vi "Read Enumerated Resources.vi"(8 "error in (no error)":errorcluster, 10 "Refresh":bool=TRUE, 11 "AbstractResourceEnumerator in":refnum<class "AbstractResourceEnumerator.lvclass">) -> (0 "error out":errorcluster, 2 "Enumerated Resources":T1[](array[typedef]), 3 "AbstractResourceEnumerator out":refnum<class "AbstractResourceEnumerator.lvclass">)   [LabVIEW 2023, in "HAF.lvlib" / "AbstractResourceEnumerator.lvclass"]
doc: "Returns the collection of resources connected to the system. The collection can be refreshed before return. If the collection is empty, resources will always be enumerated regardless of the passed indicator."
uses:
  AbstractResourceEnumerator.lvclass
  AbstractResourceEnumerator.lvclass/AbstractResourceEnumerator.ctl
  Resource Structure.ctl
  HAF.lvlib
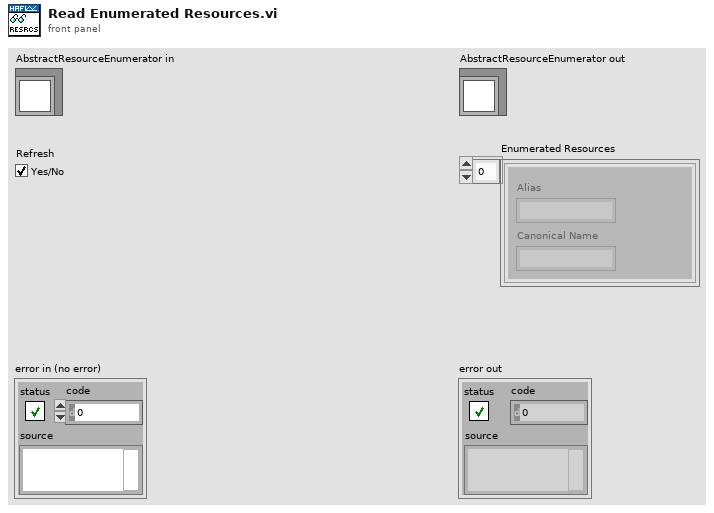
[diagram p1: front panel]
types:
  T1 = typedef "HAF.lvlib/Resource Structure.ctl" = cluster{"Alias":string, "Canonical Name":string}
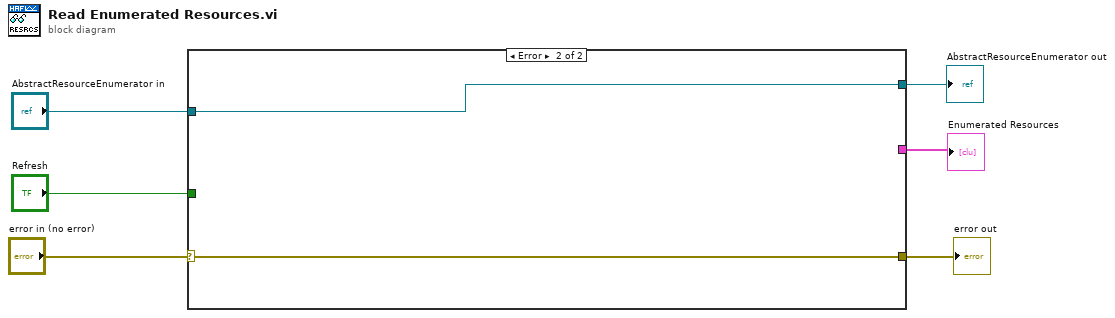
[diagram p0: block diagram]
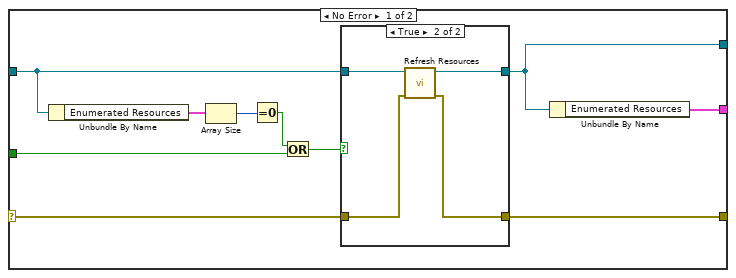
[diagram p2: hidden frame]
diagram:
  n1 = case shown="Error" "error in (no error)" {
    selector: "error in (no error)" -> [w10 w23]
    tunnel: [w9 w23] -> w5
    tunnel: [w8 w24] -> w3
    tunnel: "AbstractResourceEnumerator in" -> [w11 w24]
    tunnel: "Refresh" -> [w13 _]
    tunnel: [w7 _] -> w1
    frame No Error {
      n2 = Unbundle By Name(w11) -> ("Enumerated Resources"=w16:T1[])
      n3 = Array Size(array=w16) -> (size(s)=w15:i32)
      n4 = Equal To 0?(x=w15) -> (x = 0?=w14:bool)
      n5 = Or(x=w14, y=w13) -> (x .or. y?=w12:bool)
      n6 = case shown="True" w12 {
        tunnel: w11 -> [w18 w22]
        tunnel: w10 -> [w17 w20]
        tunnel: [w18 w21] -> w8
        tunnel: [w17 w19] -> w9
        frame False {
        }
        frame True {
          n7 = call-dynamic "Refresh Resources.vi"("error in (no error)"=w20, "AbstractResourceEnumerator in"=w22) -> ("error out"=w19:errorcluster, "AbstractResourceEnumerator out"=w21:refnum<class "AbstractResourceEnumerator.lvclass">)  [unwired: 8 in]
        }
      }
      n8 = Unbundle By Name(w8) -> ("Enumerated Resources"=w7:T1[])
    }
    frame Error {
    }
  }
  "error out" <- w5
  "AbstractResourceEnumerator out" <- w3
  "Enumerated Resources" <- w1
